vi "Test Read-Write Control Caption.vi"(8 "error in (no error)":errorcluster) -> (0 "error out":errorcluster, 3 "Pass?":bool)   [LabVIEW 2020]
uses:
  G-Unicode/Types/UTF-8 String/UTF-8 String.lvclass/UTF-8 String.ctl
  854df8bd-0e0c-48d7-82d7-b05a1342f752.vi
  G-Unicode/Dialog & User Interface/Write Control Caption (Unicode).vi/13c16a8b-00d3-486b-99f0-c83eae9facb1.vi
  G-Unicode/Dialog & User Interface/Read Control Caption (Unicode).vi/18687cfd-7198-4a8c-9005-ae619691f07e.vi
  854df8bd-0e0c-48d7-82d7-b05a1342f752.vi/3a31b270-3bb6-4c58-a256-c5fcc2c98f09.vi
  854df8bd-0e0c-48d7-82d7-b05a1342f752.vi/0ec5df2d-ef9b-4f84-a6a8-ffcedd45c4dc.vi
  G-Unicode/Private/Conversion/String as Encoded String.vi
  G-Unicode/Private/Conversion/Polymorphic VIs/String as Encoded String (UTF-8 String).vi
  G-Unicode/Private/Conversion/Encoded UTF-8 String to Encoded UTF-16LE String.vi
  G-Unicode/Private/Conversion/Text as Encoded String.vi
  G-Unicode/Private/Conversion/Polymorphic VIs/Text as Encoded String (UTF-8 String).vi
  G-Unicode/Types/UTF-8 String/Read Encoded UTF-8 String.vi
  G-Unicode/Unicode/Encode String.vi
  G-Unicode/Private/Conversion/Text to UTF-8.vi
  G-Unicode/Private/Conversion/Polymorphic VIs/Text to UTF-8 (LabVIEW String).vi
  G-Unicode/Unicode/SubVIs/UTF-16 Byte Swap.vi
  G-Unicode/Private/Conversion/UTF-8 to Text.vi
  G-Unicode/Private/Conversion/Polymorphic VIs/UTF-8 to Text (LabVIEW String).vi
  G-Unicode/Private/Conversion/Encoded UTF-16LE String to Encoded UTF-8 String.vi
  G-Unicode/Unicode/Prepend BOM.vi
  G-Unicode/Unicode/SubVIs/Byte Order Marks.vi
  G-Unicode/Unicode/Detect BOM.vi
  G-Unicode/Private/User Interface/Write Caption.vi
  G-Unicode/Private/User Interface/Read Caption.vi
  G-Unicode/Unicode/Detect String Encoding.vi
  G-Unicode/Types/UTF-8 String/UTF-8 String.lvclass
  G-Unicode/G-Unicode.lvlib
  334a5efa-86ac-4608-bd5f-4e6d67044f1d.vi
  G-Unicode/Unicode/Controls/String Encoding.ctl
panel:
  in  "OK Button":bool caption="`O}Y"
  in  "Numeric":dbl caption="Cze["
  in  "Multicolumn Listbox":i32(listbox) caption="HÅU±XÕ8Á”Æ"
  in  "Listbox":i32(listbox) caption="S0“0k0a0o0"
  in  "Table Control":string[][](table) caption="Hæ"
  in  "Menu Ring":u16(ring) caption="(\t.\t8\tM\t$\tG"
  in  "Text Ring":u16(ring) caption="ÔÙÙ"
  in  "String Array (2D)":string[][](array[string]) caption="èU"
  in  "String Array (1D)":string[](array[string]) caption="E1-('"
  in  "String":string caption="Hello"
  # "Note the dropdowns for the ring controls aren't rendered correctly, but when selected it looks OK."
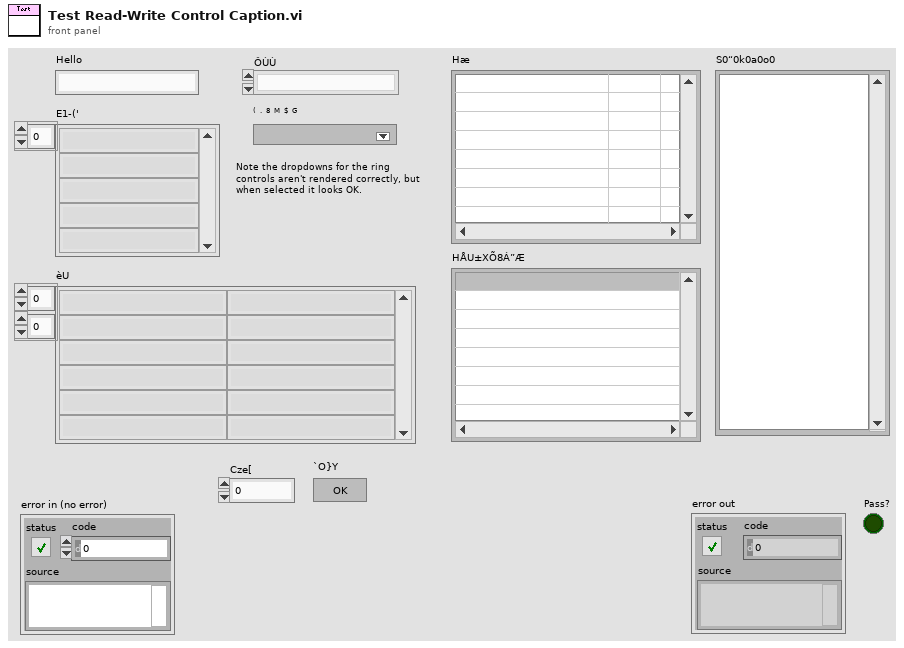
[diagram p1: front panel]
types:
  T1 = typedef "G-Unicode.lvlib/String Encoding.ctl" = enum16{"ANSI", "UTF-8", "UTF-16LE", "UTF-16BE", "Unknown"}
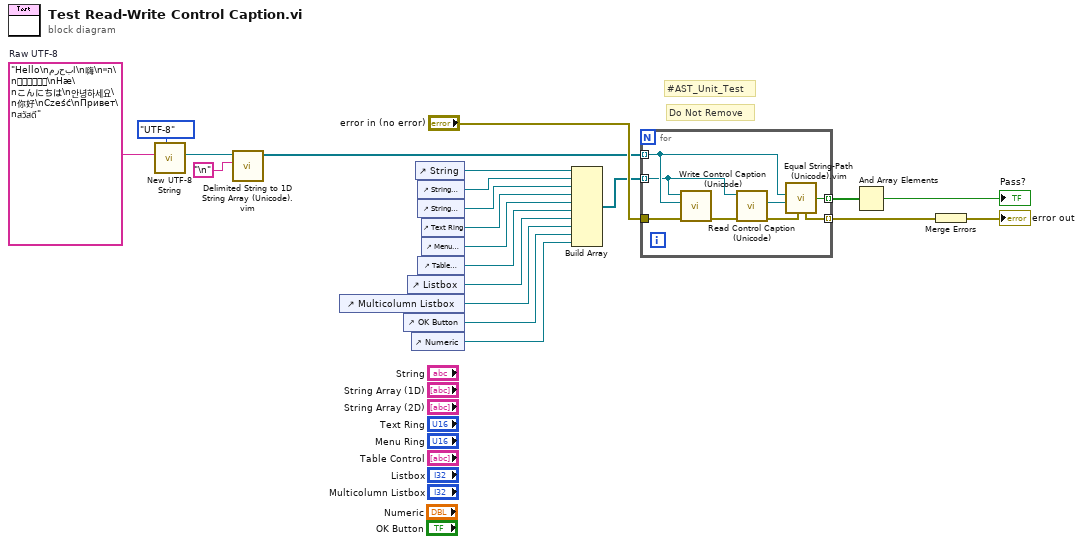
[diagram p0: block diagram]
diagram:
  w2 = "Hello\nمرحبا\n嗨\nהיי\nनमस्ते\nHæ\nこんにちは\n안녕하세요\n你好\nCześć\nПривет\nสวัสดี"  # Raw UTF-8
  # "Do Not Remove"
  # "#AST_Unit_Test"
  n1 = call "New UTF-8 String.vi"("Input Encoding (ANSI)"=String_Encoding."UTF-8", "String"=w2) -> ("UTF-8 String"=w4:refnum<class "UTF-8 String.lvclass">)  [unwired: 8 in, 1 out]
  n2 = call "Delimited String to 1D String Array (Unicode).vim"("Delimiter (tab)"="\n", "Delimited String"=w4) -> ("String Array"=w1:refnum<class "UTF-8 String.lvclass">[])  [unwired: 8 in, 1 out]
  n3 = control-ref of="Multicolumn Listbox"() -> (w13:refnum<vi>)
  n4 = control-ref of="OK Button"() -> (w9:refnum<vi>)
  n5 = control-ref of="Listbox"() -> (w14:refnum<vi>)
  n6 = control-ref of="Numeric"() -> (w8:refnum<vi>)
  n7 = control-ref of="String"() -> (w20:refnum<vi>)
  n8 = control-ref of="String Array (1D)"() -> (w19:refnum<vi>)
  n9 = control-ref of="String Array (2D)"() -> (w18:refnum<vi>)
  n10 = control-ref of="Table Control"() -> (w15:refnum<vi>)
  n11 = control-ref of="Text Ring"() -> (w17:refnum<vi>)
  n12 = control-ref of="Menu Ring"() -> (w16:refnum<vi>)
  n13 = Build Array(w20, w19, w18, w17, w16, w15, w14, w13, w9, w8) -> (w12:refnum<vi>[])
  n14 = for {
    tunnel: w12 -> [w22] mode=indexing
    tunnel: w1 -> [w23] mode=indexing
    tunnel: "error in (no error)" -> [w29]
    tunnel: [w24] -> w11 mode=indexing
    tunnel: [w26] -> w7 mode=indexing
    n15 = call "Write Control Caption (Unicode).vi"("error in"=w29, "Text"=w23, "Control Ref"=w22) -> ("error out"=w28:errorcluster)  [unwired: 8 in]
    n16 = call "Read Control Caption (Unicode).vi"("error in"=w28, "Control Ref"=w22) -> ("error out"=w25:errorcluster, "UTF-8 String"=w27:refnum<class "UTF-8 String.lvclass">)  [unwired: 8 in]
    n17 = call "Equal String-Path (Unicode).vim"("error in"=w25, "y"=w27, "x"=w23) -> ("error out"=w24:errorcluster, "Equal?"=w26:bool)  [unwired: 6 in]
  }
  n18 = And Array Elements(Boolean array=w7) -> (logical AND=→"Pass?":bool)
  n19 = Merge Errors(w11) -> (→"error out":errorcluster)
